vi "Main.vi"() -> ()   [LabVIEW 2020]
uses:
  typedef_stage_control.ctl
panel:
  in  "Cluster":T1={"Up"=FALSE, "Left"=FALSE, "Right"=FALSE, "Down"=FALSE, "Focus Down"=FALSE, "Focus Up"=FALSE, "X Step Size(um)"=6.860690000000502, "Z step size (um)"=100.0, "Y Step Size(um)"=100.0, "X Position"=0.0, "Y Position"=0.0, "Z Position"=0.0, "Enable x-axis"=FALSE, "Enable y-axis"=FALSE, "Enable z-axis"=FALSE}
  in  "Stop Button":bool
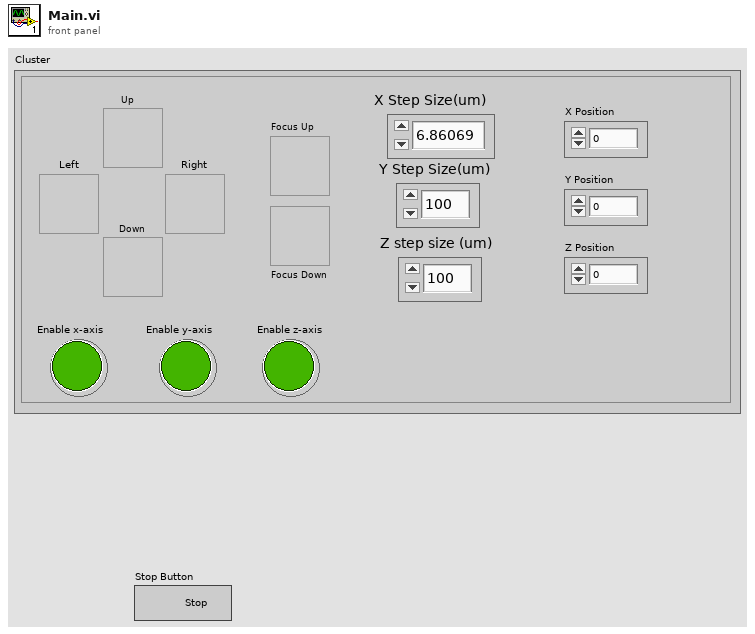
[diagram p1: front panel]
types:
  T1 = typedef "typedef_stage_control.ctl" = cluster{"Up":bool, "Left":bool, "Right":bool, "Down":bool, "Focus Down":bool, "Focus Up":bool, "X Step Size(um)":dbl, "Z step size (um)":dbl, "Y Step Size(um)":dbl, "X Position":dbl, "Y Position":dbl, "Z Position":dbl, "Enable x-axis":bool, "Enable y-axis":bool, "Enable z-axis":bool}
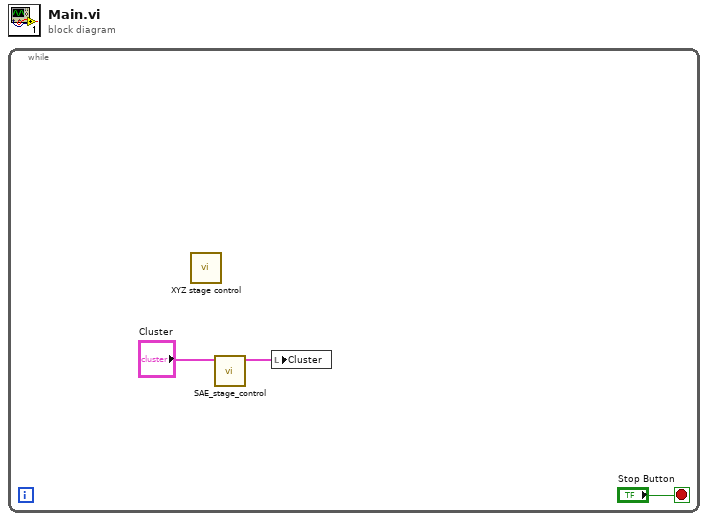
[diagram p0: block diagram]
diagram:
  n1 = while {
    stop <- "Stop Button" stop-if-true
    n2 = call "XYZ stage control.vi"() -> ()  [unwired: 12 in]
    n3 = call "SAE_stage_control.vi"("Cluster IN"="Cluster") -> ("Cluster OUT"=w1:T1)  [unwired: 7 in, 1 out]
    n4 = local write "Cluster"(w1) -> ()
  }
